vi "Boolean Array to Cluster.vi"(8 "error in":errorcluster, 11 "DIG_IO in":refnum<class "DIG_IO.lvclass">) -> (0 "error out":errorcluster, 3 "DIG_IO out":refnum<class "DIG_IO.lvclass">)   [LabVIEW 2019, in "DIG_IO.lvlib" / "DIG_IO.lvclass"]
doc: "Boolean Array data to cluster Data"
uses:
  Library/DIG_IO.lvclass
  Library/DIG_IO.lvclass/DIG_IO.ctl
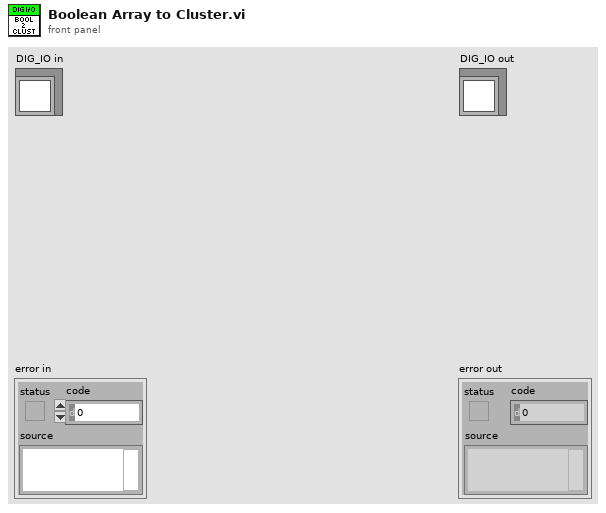
[diagram p1: front panel]
types:
  T1 = cluster{"Boolean array[0]":bool, "Boolean array[1]":bool, "Boolean array[2]":bool, "Boolean array[3]":bool, "Boolean array[4]":bool, "Boolean array[5]":bool, "Boolean array[6]":bool, "Boolean array[7]":bool}
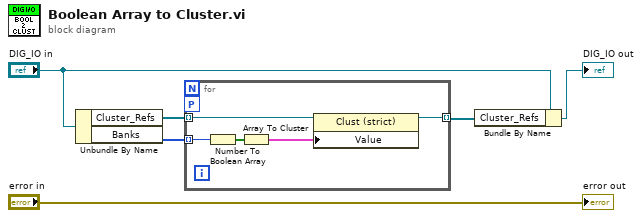
[diagram p0: block diagram]
diagram:
  n1 = Unbundle By Name("DIG_IO in") -> ("Cluster_Refs"=w3:refnum<vi>[], "Banks"=w1:u8[])
  n2 = for {
    tunnel: w3 -> [w11] mode=indexing
    tunnel: [w10] -> w2 mode=indexing
    tunnel: w1 -> [w7] mode=indexing
    workers-P: _ -> [_]
    n3 = Number To Boolean Array(number=w7) -> (Boolean array=w9:bool[])
    n4 = Array To Cluster(array=w9) -> (cluster=w8:T1)
    n5 = property class="Clust (strict)"(reference=w11, "Value"=w8) -> (reference out=w10:refnum<vi>)  [unwired: 1 in, 1 out]
  }
  n6 = Bundle By Name(cluster="DIG_IO in", "Cluster_Refs"=w2) -> (→"DIG_IO out":refnum<class "DIG_IO.lvclass">)
  "error out" <- "error in"
